vi "ReplaceSelf.vi"(0 "XRef":T12, 1 "Terms":T9, 2 "Diagram":T8, 3 "State In":T4 {"BlockNodeState"."Draw Style" items=["FunctionBlock", "ExpressVI", "Variable", "Elemental I/O", "32x32 Icon", "FunctionBlockCompact"]; "BlockNodeState"."Terminal Data"."Terminal Flags" format="%.0b"}) -> (14 "Replace Self?":T3, 15 "Reply":T1)   [LabVIEW 2017, in "NI_Robotics_Create Steering Frame.xnode"]
uses:
  <vilib>/robotics/Steering/Create Steering Frame/NI_Robotics_Create Steering Frame.xnode
  <vilib>/XNodeSupport/XNodeXNodeRef.ctl
  <vilib>/XNodeSupport/XNodeTermIDPairs.ctl
  <vilib>/XNodeSupport/XNodeTermIDPair.ctl
  <vilib>/XNodeSupport/XNodeTermRef.ctl
  <vilib>/XNodeSupport/XNodeString.ctl
  <vilib>/XNodeSupport/XNodeTopLevelDiagramRef.ctl
  <vilib>/robotics/Steering/Create Steering Frame/State.ctl
  <vilib>/BlockNodeSupport/BlockNodeState.ctl
  <vilib>/BlockNodeSupport/TerminalData.ctl
  <vilib>/picture/picture.llb/imagedata.ctl
  <vilib>/XNodeSupport/XNodeBool.ctl
  <vilib>/XNodeSupport/XNodeStringArray.ctl
  <vilib>/Utility/miscctls.llb/LVPointTypeDef.ctl
  <vilib>/XNodeSupport/NI_XNodeSupport.lvlib
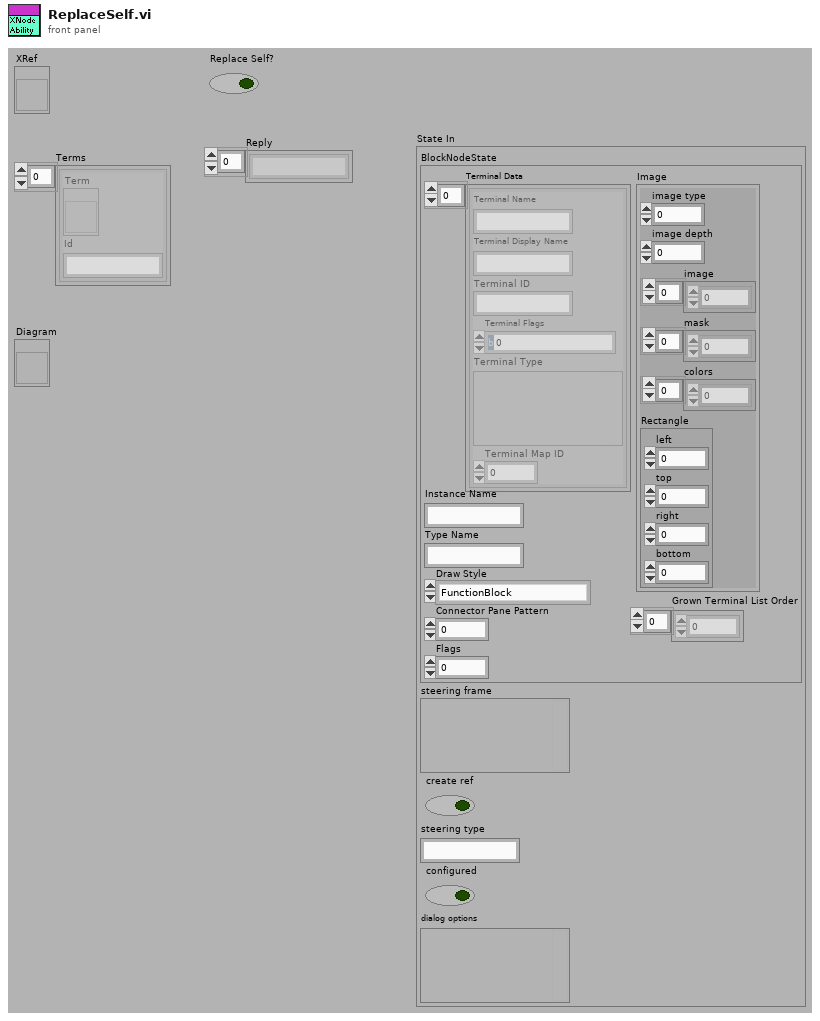
[diagram p1: front panel]
types:
  T1 = typedef "NI_XNodeSupport.lvlib/XNodeStringArray.ctl" = T2[]
  T2 = typedef "NI_XNodeSupport.lvlib/XNodeString.ctl" = string
  T3 = typedef "NI_XNodeSupport.lvlib/XNodeBool.ctl" = bool
  T4 = typedef "NI_Robotics_Create Steering Frame.xnode/State.ctl" = cluster{"BlockNodeState":T5, "steering frame":variant, "create ref":bool, "steering type":string, "configured":bool, "dialog options":variant}
  T5 = typedef "BlockNodeState.ctl" = cluster{"Terminal Data":T6[], "Instance Name":string, "Type Name":string, "Draw Style":i32, "Connector Pane Pattern":i32, "Flags":i32, "Grown Terminal List Order":i32[], "Image":T7}
  T6 = typedef "TerminalData.ctl" = cluster{"Terminal Name":string, "Terminal Display Name":string, "Terminal ID":string, "Terminal Flags":i32, "Terminal Type":variant, "Terminal Map ID":i32}
  T7 = typedef "imagedata.ctl" = cluster{"image type":i32, "image depth":i32, "image":u8[], "mask":u8[], "colors":u32[], "Rectangle":cluster{"left":i16, "top":i16, "right":i16, "bottom":i16}}
  T8 = typedef "NI_XNodeSupport.lvlib/XNodeTopLevelDiagramRef.ctl" = refnum<vi>
  T9 = typedef "NI_XNodeSupport.lvlib/XNodeTermIDPairs.ctl" = T10[]
  T10 = typedef "NI_XNodeSupport.lvlib/XNodeTermIDPair.ctl" = cluster{"Term":T11, "Id":T2}
  T11 = typedef "NI_XNodeSupport.lvlib/XNodeTermRef.ctl" = refnum<vi>
  T12 = typedef "NI_XNodeSupport.lvlib/XNodeXNodeRef.ctl" = refnum<vi>
  T13 = typedef "LVPointTypeDef.ctl" = cluster{"Horizontal":i16, "Vertical":i16}
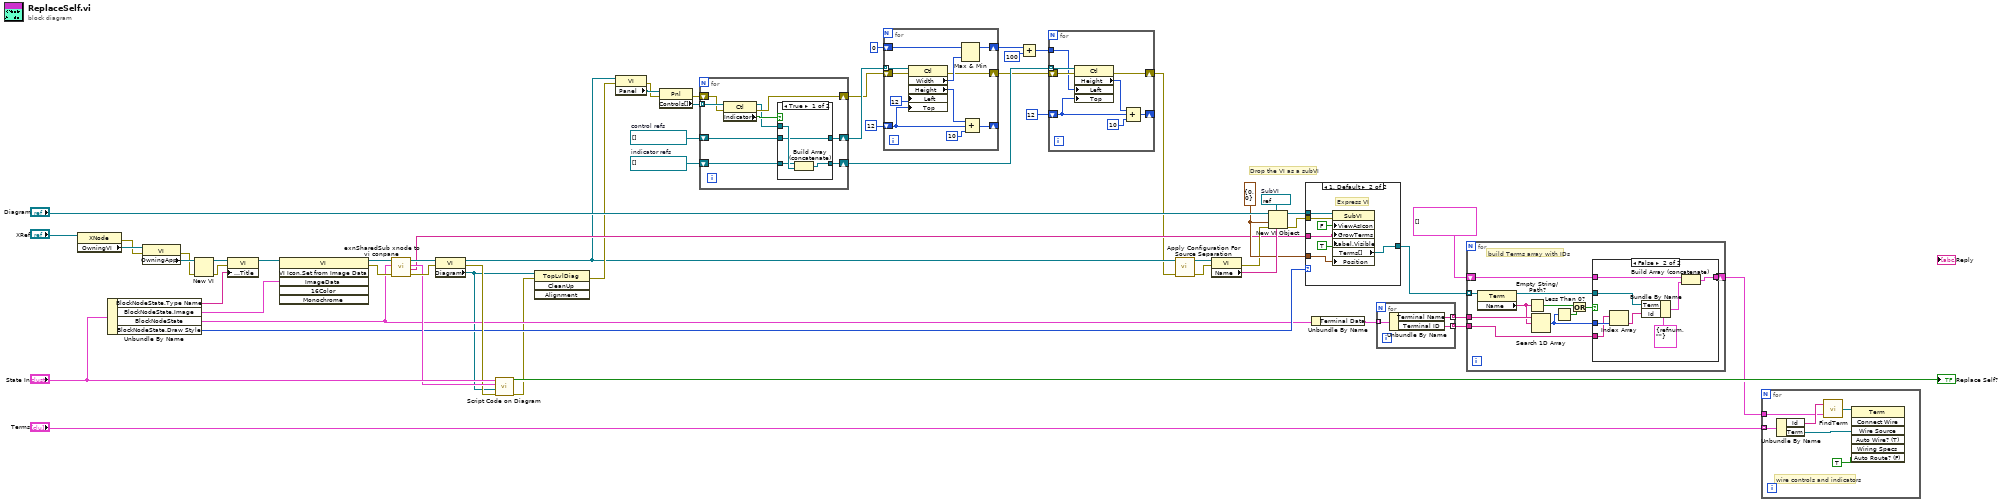
[diagram p0: block diagram]
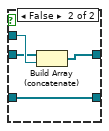
[diagram p2: hidden frame]
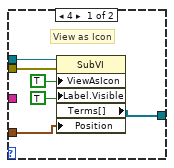
[diagram p4: hidden frame]
diagram:
  w16 = refnum<vi>[] []  # indicator refs
  w17 = refnum<vi>[] []  # control refs
  w33 = T13 {"Horizontal"=0, "Vertical"=0} ("relative position/next to refnum")
  w39 = refnum<vi> refnum  # SubVI
  # "Drop the VI as a subVI"
  n1 = property class="XNode"(reference="XRef") -> (error out=w52:errorcluster, "OwningVI"=w53:refnum<vi>)  [unwired: 1 in, 1 out]
  n2 = Unbundle By Name("State In") -> ("BlockNodeState.Type Name"=w44:string, "BlockNodeState.Image"=w49:T7, "BlockNodeState"=w30:T5, "BlockNodeState.Draw Style"=w34:i32)
  n3 = property class="VI"(reference=w53, error in=w52) -> (error out=w50:errorcluster, "OwningApp"=w51:refnum<vi>)  [unwired: 1 out]
  n4 = New VI(8:w50, 11:w51) -> (0:w45:errorcluster, 3:w47:refnum<vi>)  [unwired: 5 out]
  n5 = property class="VI"(reference=w47, error in=w45, "Front Panel.Title"=w44) -> (reference out=w46:refnum<vi>)  [unwired: 1 out]
  n6 = invoke class="VI" method="VI Icon.Set from Image Data"(reference=w46, "ImageData"=w49) -> (reference out=w48:refnum<vi>, error out=w43:errorcluster)  [unwired: 4 in, 4 out]
  n7 = call <vilib>:"exnSharedSub xnode to vi conpane.vi"("error in (no error)"=w43, "BlockNodeState"=w30, "VI Refnum"=w48) -> ("error out"=w41:errorcluster, "GrownTerms"=w31:string[], "Terms"=w40:T9, "VI Refnum out"=w42:refnum<vi>)  [unwired: 5 out]
  n8 = property class="VI"(reference=w42, error in=w41) -> (reference out=w4:refnum<vi>, error out=w37:errorcluster, "Diagram"=w24:refnum<vi>)
  n9 = call <vilib>:"Script Code on Diagram.vi"("error in (no error)"=w37, "diagram"=w24, "Terms"=w40, "State In"="State In") -> ("error out"=w23:errorcluster, "generated?"=→"Replace Self?":bool)  [unwired: 6 in]
  n10 = invoke class="TopLvlDiag" method="CleanUp"(reference=w24, error in=w23) -> (error out=w5:errorcluster)  [unwired: 2 in, 3 out]
  n11 = property class="VI"(reference=w4, error in=w5) -> (error out=w20:errorcluster, "Panel"=w21:refnum<vi>)  [unwired: 1 out]
  n12 = property class="Pnl"(reference=w21, error in=w20) -> (error out=w18:errorcluster, "Controls[]"=w19:refnum<vi>[])  [unwired: 1 out]
  n13 = for {
    tunnel: w19 -> [w67] mode=indexing
    shift-right: [w64] -> w11
    shift-left: w18 -> [w66]
    shift-right: [w59] -> w15
    shift-left: w17 -> [w62]
    shift-right: [w60] -> w12
    shift-left: w16 -> [w61]
    n14 = property class="Ctl"(reference=w67, error in=w66) -> (reference out=w63:refnum<vi>, error out=w64:errorcluster, "Indicator"=w65:bool)
    n15 = case shown="True" w65 {
      tunnel: w63 -> [w71 w75]
      tunnel: w62 -> [w68 w74]
      tunnel: w61 -> [w70 w72]
      tunnel: [w69 w72] -> w60
      tunnel: [w68 w73] -> w59
      frame True {
        n16 = Build Array (concatenate)(w70, w71) -> (w69:refnum<vi>[])
      }
      frame False {
        n17 = Build Array (concatenate)(w74, w75) -> (w73:refnum<vi>[])
      }
    }
  }
  n18 = for {
    tunnel: w15 -> [w86] mode=indexing
    shift-right: [w84] -> w8
    shift-left: u32 0 -> [w83]
    shift-right: [w79] -> _
    shift-left: u32 12 ("Position:Top") -> [w80]
    shift-right: [w76] -> w10
    shift-left: w11 -> [w77]
    n19 = property class="Ctl"(reference=w86, error in=w77, "Left"=12 ("Position:Left"), "Top"=w80) -> (error out=w76:errorcluster, "Width"=w85:u32, "Height"=w81:u32)  [unwired: 1 out]
    n20 = Max & Min(x=w83, y=w85) -> (max(x,y)=w84:u32)  [unwired: 1 out]
    n21 = Compound Arithmetic op=ADD(w81, w80, u32 10 ("value")) -> (w79:u32)
  }
  n22 = Add(x=w8, y=u32 100) -> (x+y=w7:u32)
  n23 = for {
    tunnel: w12 -> [w94] mode=indexing
    shift-right: [w91] -> w2
    shift-left: w10 -> [w93]
    tunnel: w7 -> [w92]
    shift-right: [w88] -> _
    shift-left: u32 12 ("Position:Top") -> [w89]
    n24 = property class="Ctl"(reference=w94, error in=w93, "Left"=w92, "Top"=w89) -> (error out=w91:errorcluster, "Height"=w87:u32)  [unwired: 1 out]
    n25 = Compound Arithmetic op=ADD(w87, w89, u32 10 ("value")) -> (w88:u32)
  }
  n26 = call <vilib>:"Apply Configuration For Source Separation.vi"("error in (no error)"=w2, "VI in"=w4) -> ("error out"=w1:errorcluster, "VI out"=w3:refnum<vi>)  [unwired: 8 in]
  n27 = property class="VI"(reference=w3, error in=w1) -> (error out=w32:errorcluster, "Name"=w38:string)  [unwired: 1 out]
  n28 = New VI Object(vi object class=w39, owner refnum="Diagram", position/next to=w33, 6:w38, 8:w32) -> (object refnum=w36:refnum<vi>, 0:w35:errorcluster)  [unwired: 3 out]
  n29 = case shown="1, Default" w34 {
    tunnel: [w100 w107] -> w26
    tunnel: w36 -> [w99 w106]
    tunnel: w33 -> [w98 w105]
    tunnel: w31 -> [_ w104]
    tunnel: w35 -> [w97 w103]
    frame 4 {
      # "View as Icon"
      n30 = property class="SubVI"(reference=w99, error in=w97, "ViewAsIcon"=TRUE ("View As Icon"), "Label.Visible"=TRUE, "Position"=w98) -> ("Terms[]"=w100:refnum<vi>[])  [unwired: 2 out]
    }
    frame 1, Default {
      # "Express VI"
      n31 = property class="SubVI"(reference=w106, error in=w103, "ViewAsIcon"=FALSE ("View As Icon"), "GrowTerms"=w104, "Label.Visible"=TRUE, "Position"=w105) -> ("Terms[]"=w107:refnum<vi>[])  [unwired: 2 out]
    }
  }
  n32 = Unbundle By Name(w30) -> ("Terminal Data"=w29:T6[])
  n33 = for {
    tunnel: w29 -> [w110] mode=indexing
    tunnel: [w109] -> w27 mode=indexing
    tunnel: [w108] -> w28 mode=indexing
    n34 = Unbundle By Name(w110) -> ("Terminal Name"=w109:string, "Terminal ID"=w108:string)
  }
  n35 = for {
    tunnel: w26 -> [w121] mode=indexing
    tunnel: w27 -> [w120]
    tunnel: w28 -> [w112]
    shift-right: [w117] -> w25
    shift-left: T9 [] ("Code Gen Term Array") -> [w118]
    # "build Terms array with IDs"
    n36 = property class="Term"(reference=w121) -> (reference out=w119:refnum<vi>, "Name"=w111:string)  [unwired: 1 in, 1 out]
    n37 = Empty String/Path?(string/path=w111) -> (empty?=w116:bool)
    n38 = Search 1D Array(1D array=w120, element=w111) -> (index of element=w115:i32)  [unwired: 1 out]
    n39 = Less Than 0?(x=w115) -> (x < 0?=w113:bool)
    n40 = Or(x=w116, y=w113) -> (x .or. y?=w114:bool)
    n41 = case shown="False" w114 {
      tunnel: w119 -> [_ w130]
      tunnel: w118 -> [w122 w127]
      tunnel: [w122 w126] -> w117
      tunnel: w115 -> [_ w125]
      tunnel: w112 -> [_ w124]
      frame True {
      }
      frame False {
        n42 = Index Array(array=w124, index=w125) -> (element=w129:string)
        n43 = Bundle By Name(cluster=T10 {"Term"=refnum, "Id"=""} ("Code Gen Term"), "Term"=w130, "Id"=w129) -> (w128:T10)
        n44 = Build Array (concatenate)(w127, w128) -> (w126:T9)
      }
    }
  }
  n45 = for {
    tunnel: "Terms" -> [w135] mode=indexing
    tunnel: w25 -> [w132]
    # "wire controls and indicators"
    n46 = Unbundle By Name(w135) -> ("Id"=w133:T2, "Term"=w134:T11)
    n47 = call <vilib>:"FindTerm.vi"("Terms"=w132, "String"=w133) -> ("Term"=w131:refnum<vi>)
    n48 = invoke class="Term" method="Connect Wire"(reference=w131, "Wire Source"=w134, "Auto Route? (F)"=TRUE) -> ()  [unwired: 4 in, 7 out]
  }
